vi "Pipe Var Intf - Test Write Timeout.vi"() -> ()   [LabVIEW 2020, in "GOLPI library.lvlib"]
uses:
  GOLPI library.lvlib
panel:
  out "available bytes":u32
  in  "write block size (10k)":i32=10000
  in  "timeout [s]":dbl=3.0
  out "read bytes":u32
  in  "bytes to read (0)":i32
  in  "btn read":bool
  in  "data size":i32=100000
  out "handle":i32
  in  "btn stop client":bool
  in  "btn close":bool
  out "error out 2":errorcluster
  in  "btn open":bool
  in  "pipe name in (leave empty to generate random name)":string="\\\\.\\Pipe\\GOLPI_Variable_Pipe"
  out "error out":errorcluster
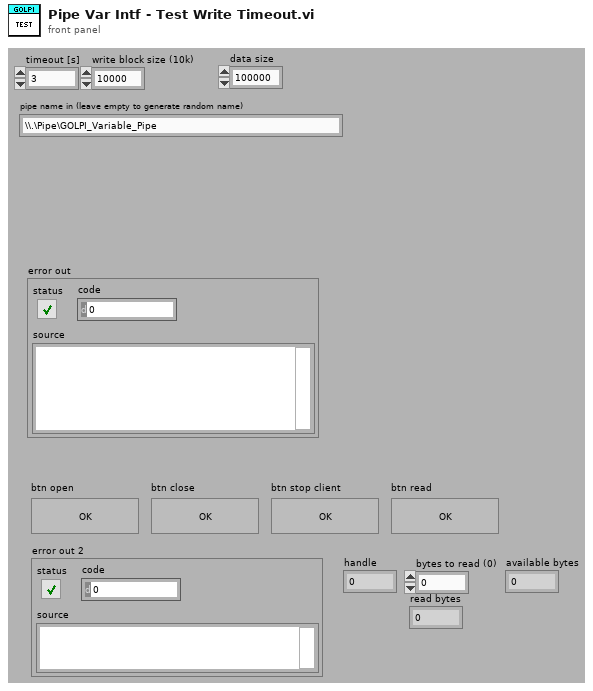
[diagram p1: front panel]
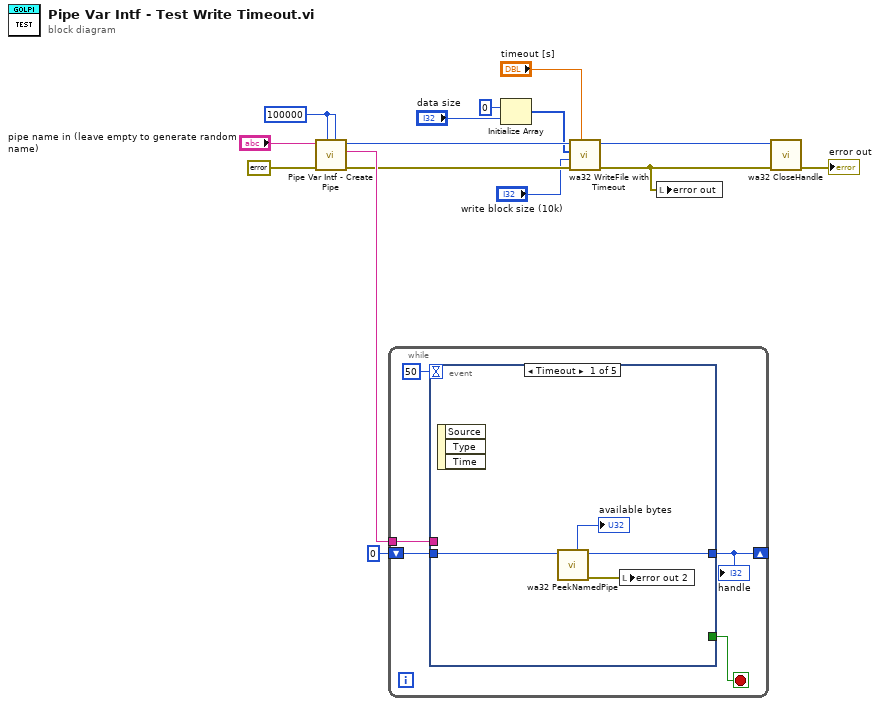
[diagram p0: block diagram]
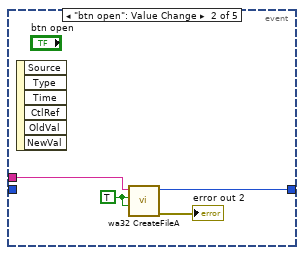
[diagram p2: hidden frame]
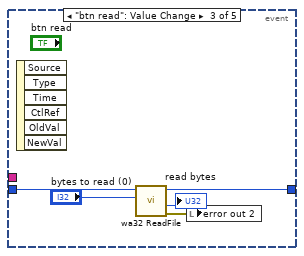
[diagram p3: hidden frame]
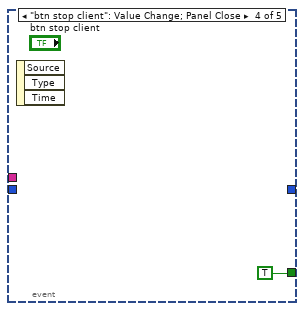
[diagram p4: hidden frame]
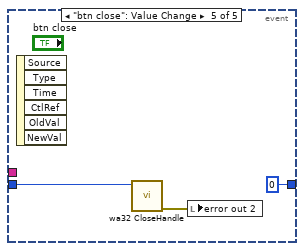
[diagram p5: hidden frame]
diagram:
  w10 = u32 100000 ("inBufferSize (256k)")
  n1 = call "Pipe Var Intf - Create Pipe.vi"("outBufferSize (256k)"=w10, "inBufferSize (256k)"=w10, "error in (no error)"=errorcluster {"status"=FALSE, "code"=0, "source"=""} ("error out"), "pipe name in (leave empty to generate random name)"="pipe name in (leave empty to generate random name)") -> ("error out"=w7:errorcluster, "pipe name out"=w11:string, "pipe handle out"=w6:i32)  [unwired: 5 in]
  n2 = while {
    shift-right: [w20] -> _
    shift-left: 0 ("handle") -> [w19]
    tunnel: w11 -> [w18]
    stop <- w17 stop-if-true
    n3 = event shown="[0] Timeout" {
      selector: _ -> [_ _ _ _ _]
      dyn-events: _ -> [_ _ _ _ _]
      timeout: 50 -> [_ _ _ _ _]
      tunnel: [w23 w27 w32 _ 0 ("handle")] -> w20
      tunnel: w19 -> [w24 _ w33 _ w37]
      tunnel: w18 -> [_ w26 _ _ _]
      tunnel: [_ _ _ TRUE _] -> w17
      event Timeout {
        n4 = event-data() -> ()  [unwired: 1 in, 3 out]
        n5 = call "wa32 PeekNamedPipe.vi"("handle"=w24) -> ("error out"=w22:errorcluster, "handle out"=w23:i32, "available bytes"=→"available bytes":u32)  [unwired: 5 in, 3 out]
        n6 = local write "error out 2"(w22) -> ()
      }
      event "btn open": Value Change {
        w25 = TRUE ("read")
        n7 = event-data() -> ()  [unwired: 1 in, 6 out]
        n8 = call "wa32 CreateFileA.vi"("write"=w25, "read"=w25, "file path"=w26) -> ("error out"=→"error out 2":errorcluster, "handle"=w27:i32)  [unwired: 7 in]
      }
      event "btn read": Value Change {
        n9 = event-data() -> ()  [unwired: 1 in, 6 out]
        n10 = call "wa32 ReadFile.vi"("bytes to read (0)"="bytes to read (0)", "handle"=w33) -> ("error out"=w31:errorcluster, "read bytes"=→"read bytes":u32, "handle out"=w32:i32)  [unwired: 5 in, 2 out]
        n11 = local write "error out 2"(w31) -> ()
      }
      event "btn stop client": Value Change; Panel Close {
        n12 = event-data() -> ()  [unwired: 1 in, 3 out]
      }
      event "btn close": Value Change {
        n13 = event-data() -> ()  [unwired: 1 in, 6 out]
        n14 = call "wa32 CloseHandle.vi"("handle"=w37) -> ("error out"=w35:errorcluster)  [unwired: 10 in]
        n15 = local write "error out 2"(w35) -> ()
      }
    }
    "handle" <- w20
  }
  n16 = Initialize Array(u8 0 ("element"), "data size") -> (w3:u8[])
  n17 = call "wa32 WriteFile with Timeout.vi"("timeout [s]"="timeout [s]", "error in (no error)"=w7, "write block size (10k)"="write block size (10k)", "data"=w3, "pipe handle"=w6) -> ("error out"=w4:errorcluster, "pipe handle out"=w5:i32)  [unwired: 4 in, 1 out]
  n18 = local write "error out"(w4) -> ()
  n19 = call "wa32 CloseHandle.vi"("error in"=w4, "handle"=w5) -> ("error out"=→"error out":errorcluster)  [unwired: 9 in]
